vi "Set Main GUI for Different Acquire States.vi"(8 "Error In":errorcluster, 11 "Scan Type [Out]":T1) -> (0 "Error Out":errorcluster)   [LabVIEW 2014]
uses:
  Controls/ScanType.ctl
  Controls/GUI Module Actions.ctl
  Controls/GUI Types.ctl
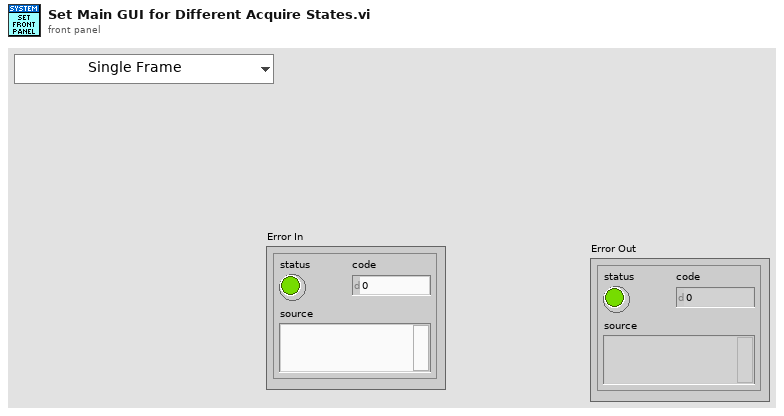
[diagram p1: front panel]
types:
  T1 = typedef "ScanType.ctl" = enum16{"Single Frame", "Continuous Frame", "ROI Line", "Vibratome", "Mosaic", "Mosaic + Slice"}
  T2 = typedef "GUI Module Actions.ctl" = enum16{"Init", "Open Front Panel", "Hide All Front Panels", "Close Front Panel", "Uninit"}
  T3 = typedef "GUI Types.ctl" = enum16{"Mosaic GUI", "Vibratome GUI"}
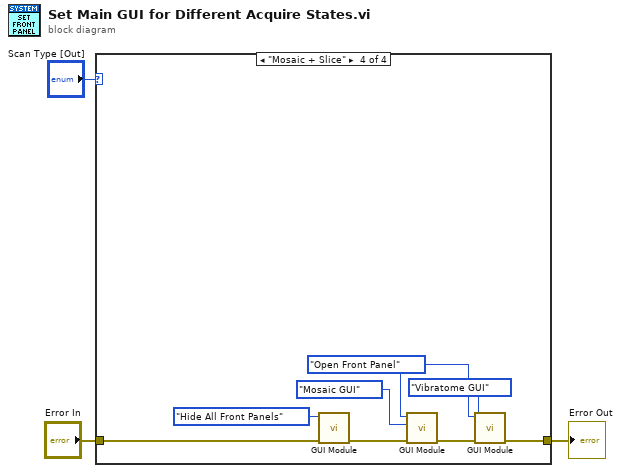
[diagram p0: block diagram]
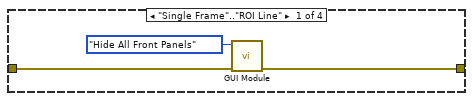
[diagram p2: hidden frame]
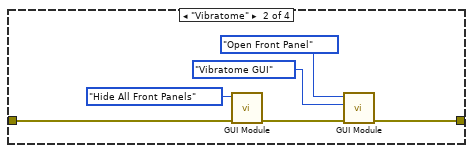
[diagram p3: hidden frame]
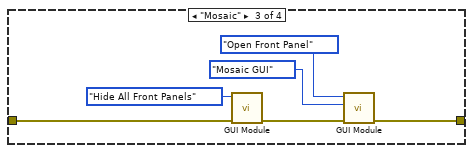
[diagram p4: hidden frame]
diagram:
  n1 = case shown="\"Mosaic + Slice\"" "Scan Type [Out]" {
    tunnel: "Error In" -> [w6 w12 w18 w26]
    tunnel: [w5 w9 w15 w21] -> w1
    frame "Single Frame".."ROI Line" {
      n2 = call "GUI Module.vi"("Error In"=w6, "GUI Actions"=GUI_Module_Actions."Hide All Front Panels") -> ("Error Out"=w5:errorcluster)  [unwired: 9 in]
    }
    frame "Vibratome" {
      n3 = call "GUI Module.vi"("Error In"=w12, "GUI Actions"=GUI_Module_Actions."Hide All Front Panels") -> ("Error Out"=w11:errorcluster)  [unwired: 9 in]
      n4 = call "GUI Module.vi"("Error In"=w11, "GUI Types"=GUI_Types."Vibratome GUI", "GUI Actions"=GUI_Module_Actions."Open Front Panel") -> ("Error Out"=w9:errorcluster)  [unwired: 8 in]
    }
    frame "Mosaic" {
      n5 = call "GUI Module.vi"("Error In"=w18, "GUI Actions"=GUI_Module_Actions."Hide All Front Panels") -> ("Error Out"=w17:errorcluster)  [unwired: 9 in]
      n6 = call "GUI Module.vi"("Error In"=w17, "GUI Types"=GUI_Types."Mosaic GUI", "GUI Actions"=GUI_Module_Actions."Open Front Panel") -> ("Error Out"=w15:errorcluster)  [unwired: 8 in]
    }
    frame "Mosaic + Slice" {
      w20 = GUI_Module_Actions."Open Front Panel" ("GUI Actions")
      n7 = call "GUI Module.vi"("Error In"=w26, "GUI Actions"=GUI_Module_Actions."Hide All Front Panels") -> ("Error Out"=w25:errorcluster)  [unwired: 9 in]
      n8 = call "GUI Module.vi"("Error In"=w25, "GUI Types"=GUI_Types."Mosaic GUI", "GUI Actions"=w20) -> ("Error Out"=w23:errorcluster)  [unwired: 8 in]
      n9 = call "GUI Module.vi"("Error In"=w23, "GUI Types"=GUI_Types."Vibratome GUI", "GUI Actions"=w20) -> ("Error Out"=w21:errorcluster)  [unwired: 8 in]
    }
  }
  "Error Out" <- w1
